vi "Login.vi"(8 "error in (no error)":errorcluster, 11 "session":T1) -> (0 "error out":errorcluster)   [LabVIEW 2013, in "libssh2_integration_tests.lvlib"]
uses:
  libssh2_integration_tests.lvlib
  libssh2/Session Refnum.ctl
  libssh2/libssh2.lvlib
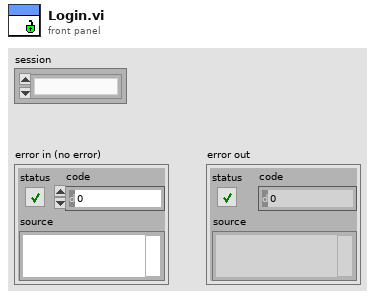
[diagram p1: front panel]
types:
  T1 = typedef "libssh2.lvlib/Session Refnum.ctl" = refnum<k1>
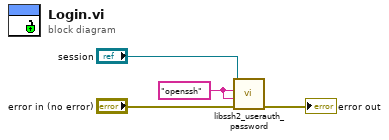
[diagram p0: block diagram]
diagram:
  w4 = "openssh" ("username")
  n1 = call "libssh2_userauth_password.vi"("error in (no error)"="error in (no error)", "password"=w4, "username"=w4, "session"="session") -> ("error out"=→"error out":errorcluster)  [unwired: 7 in]
